vi "U8 normalization.vi"(1 "Max":dbl, 2 "Input":dbl[](array[numeric])) -> (0 "Output":u8[](array[numeric]))   [LabVIEW 2012]
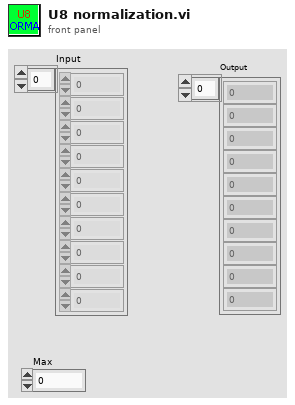
[diagram p1: front panel]
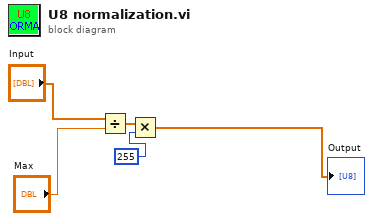
[diagram p0: block diagram]
diagram:
  n1 = Divide(x="Input", y="Max") -> (x/y=w3:dbl[])
  n2 = Multiply(x=w3, y=255) -> (x*y=→"Output":dbl[])
